vi "SCPI_2commandSender.vi"() -> ()   [LabVIEW 2016]
uses:
  <vilib>/Instr/_visa.llb/VISA Configure Serial Port (Instr).vi
panel:
  in  "Enable Termination\nChar (T)":bool=TRUE
  in  "baud rate (9600)":u32=19200
  in  "VISA resource name":refnum<visa-resource-name>
  in  "do2ndCMD":bool
  in  "cmd 2":string
  in  "Query":bool
  out "error out":errorcluster
  out "return count":u32
  out "read buffer":string
  in  "write buffer":string
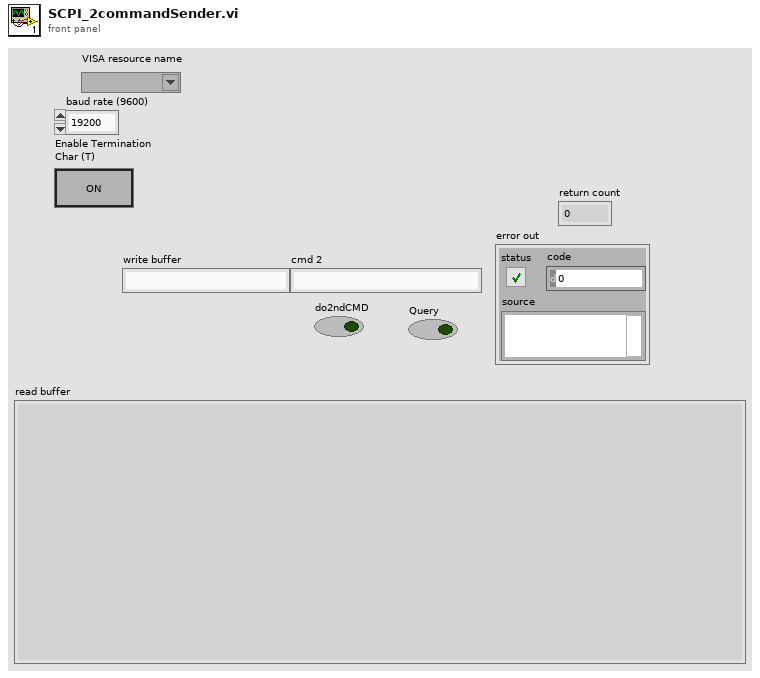
[diagram p1: front panel]
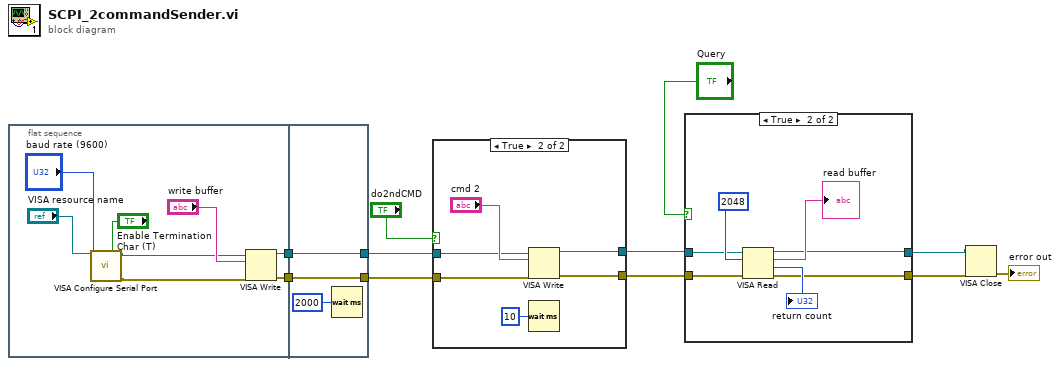
[diagram p0: block diagram]
diagram:
  n1 = flat-sequence {
    tunnel: [w18] -> w2
    tunnel: [w17] -> w1
    tunnel: [w21] -> w6
    tunnel: [w22] -> w7
    tunnel: w2 -> [w22]
    tunnel: w1 -> [w21]
    frame #0 {
      n2 = call-poly "VISA Configure Serial Port"("VISA resource name"="VISA resource name", "Enable Termination\nChar (T)"="Enable Termination\nChar (T)", "baud rate (9600)"="baud rate (9600)") -> ("VISA resource name out"=w16:refnum<visa-resource-name>, "error out"=w15:errorcluster)  [unwired: 11 in]
      n3 = VISA Write(VISA resource name=w16, write buffer="write buffer", error in (no error)=w15) -> (VISA resource name out=w18:refnum<visa-resource-name>, error out=w17:errorcluster)  [unwired: 1 out]
    }
    frame #1 {
      n4 = Wait (ms)(milliseconds to wait=u32 2000) -> ()  [unwired: 1 out]
    }
  }
  n5 = case shown="True" "do2ndCMD" {
    tunnel: w7 -> [w24 w29]
    tunnel: w6 -> [w23 w28]
    tunnel: [w23 w27] -> w5
    tunnel: [w24 w26] -> w4
    frame False {
    }
    frame True {
      n6 = VISA Write(VISA resource name=w29, write buffer="cmd 2", error in (no error)=w28) -> (VISA resource name out=w26:refnum<visa-resource-name>, error out=w27:errorcluster)  [unwired: 1 out]
      n7 = Wait (ms)(milliseconds to wait=u32 10) -> ()  [unwired: 1 out]
    }
  }
  n8 = case shown="True" "Query" {
    tunnel: w4 -> [w32 w36]
    tunnel: w5 -> [w31 w35]
    tunnel: [w32 w34] -> w9
    tunnel: [w31 w33] -> w8
    frame False {
    }
    frame True {
      n9 = VISA Read(VISA resource name=w36, byte count=u32 2048, error in (no error)=w35) -> (VISA resource name out=w34:refnum<visa-resource-name>, read buffer=→"read buffer":string, return count=→"return count":u32, error out=w33:errorcluster)
    }
  }
  n10 = VISA Close(VISA resource name=w9, error in (no error)=w8) -> (error out=→"error out":errorcluster)
